vi "Facade.vi"(0 "Data In":T4, 2 "Display State In":T2, 3 "Container State":T3) -> (6 "Data Out":T4, 7 "Display State Out":T2, 8 "Action":T1)   [LabVIEW 2015, in "FM Sweep.xctl"]
uses:
  FM Sweep.xctl
  <vilib>/_xctls/Action.ctl
  <vilib>/_xctls/XControlSupport.lvlib
  Classes/Waveforms/FM Sweep/FM Sweep.lvclass
  <vilib>/_xctls/Container State.ctl
  Data.vi
  State.vi
panel:
  in  "mode":enum16{"Linear", "Log"}(ring)
  in  "ramp constant":bool caption="Hold freq const during ramp"
  in  "Fmax (Hz)":dbl
  in  "Fmin (Hz)":dbl
  in  "Rate":dbl caption="Rate (oct/s)"
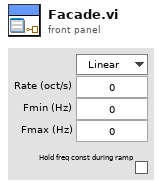
[diagram p1: front panel]
types:
  T1 = typedef "XControlSupport.lvlib/Action.ctl" = cluster{"Data Changed?":bool, "State Changed?":bool, "Action Name":string}
  T2 = typedef "FM Sweep.xctl/State.vi" = cluster{"Numeric":dbl}
  T3 = typedef "XControlSupport.lvlib/Container State.ctl" = cluster{"Indicator?":bool, "Run Mode?":bool, " Refnum":refnum<vi>}
  T4 = typedef "FM Sweep.xctl/Data.vi" = refnum<class "FM Sweep.lvclass">
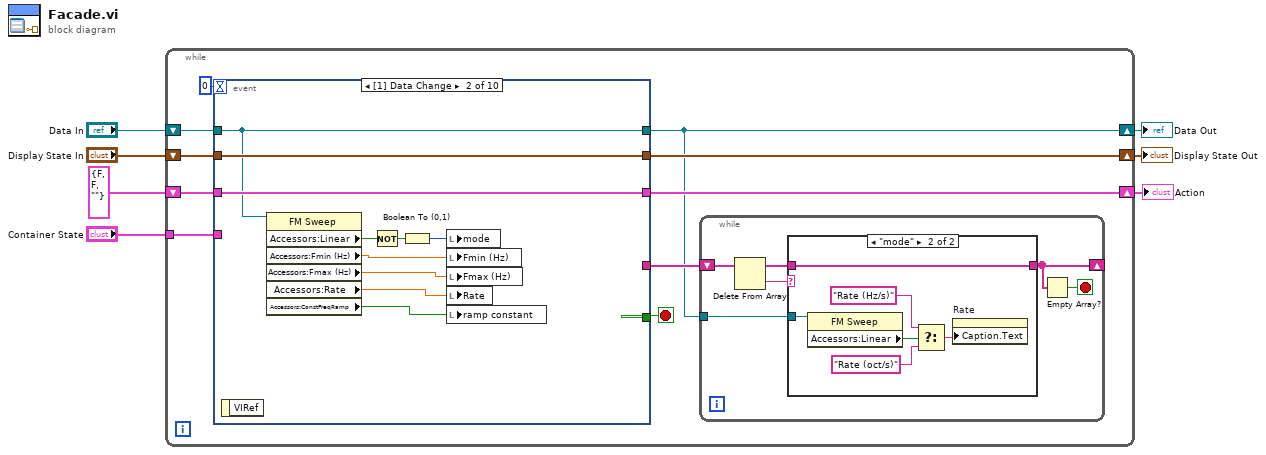
[diagram p0: block diagram]
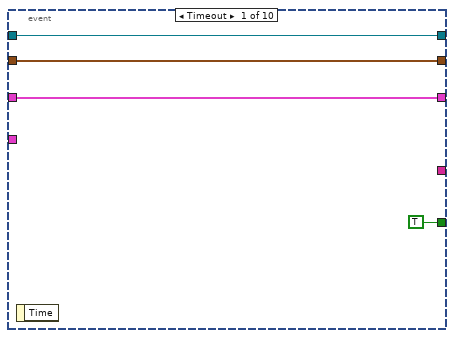
[diagram p3: hidden frame]
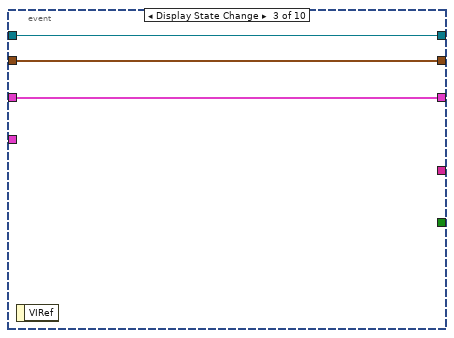
[diagram p4: hidden frame]
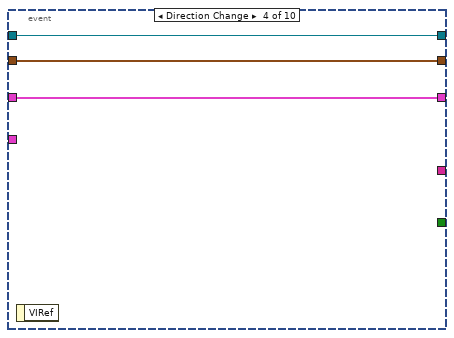
[diagram p5: hidden frame]
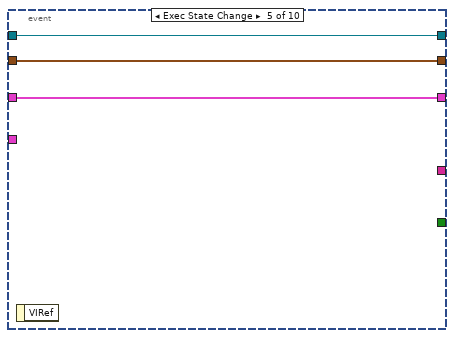
[diagram p6: hidden frame]
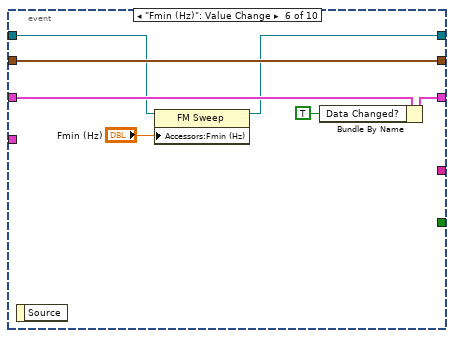
[diagram p7: hidden frame]
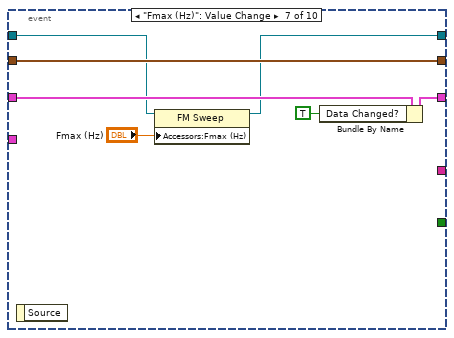
[diagram p8: hidden frame]
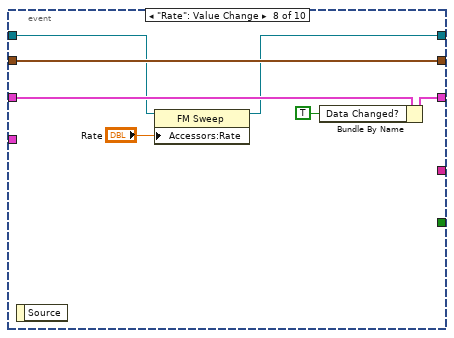
[diagram p9: hidden frame]
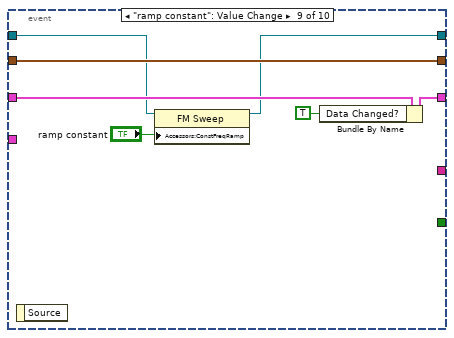
[diagram p10: hidden frame]
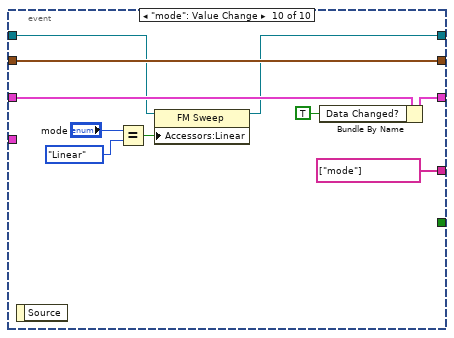
[diagram p11: hidden frame]
diagram:
  n1 = while {
    shift-right: [w16] -> w4
    shift-left: "Display State In" -> [w17]
    tunnel: "Container State" -> [w13]
    shift-right: [w8] -> w7
    shift-left: "Data In" -> [w12]
    shift-right: [w10] -> w2
    shift-left: T1 {"Data Changed?"=FALSE, "State Changed?"=FALSE, "Action Name"=""} ("Action") -> [w11]
    stop <- w15 stop-if-true
    n2 = event shown="[1] Data Change" {
      selector: _ -> [_ _ _ _ _ _ _ _ _ _]
      dyn-events: _ -> [_ _ _ _ _ _ _ _ _ _]
      timeout: 0 -> [_ _ _ _ _ _ _ _ _ _]
      tunnel: w17 -> [w32 w44 w47 w50 w53 w60 w67 w74 w81 w91]
      tunnel: [w32 w44 w47 w50 w53 w60 w67 w74 w81 w91] -> w16
      tunnel: [TRUE _ _ _ _ _ _ _ _ _] -> w15
      tunnel: w13 -> [_ _ _ _ _ _ _ _ _ _]
      tunnel: w12 -> [w31 w42 w46 w49 w52 w58 w65 w72 w79 w89]
      tunnel: [w31 w42 w46 w49 w52 w57 w64 w71 w78 w88] -> w8
      tunnel: [w33 w43 w45 w48 w51 w56 w63 w70 w77 w87] -> w10
      tunnel: w11 -> [w33 w43 w45 w48 w51 w59 w66 w73 w80 w90]
      tunnel: [_ _ _ _ _ _ _ _ _ string[] ["mode"]] -> w9
      event Timeout {
        n3 = event-data() -> ()  [unwired: 1 in, 1 out]
      }
      event Data Change {
        n4 = event-data() -> ()  [unwired: 1 in, 1 out]
        n5 = property class="FM Sweep"(reference=w42) -> ("Accessors:Linear"=w41:bool, "Accessors:Fmin (Hz)"=w38:dbl, "Accessors:Fmax (Hz)"=w37:dbl, "Accessors:Rate"=w36:dbl, "Accessors:ConstFreqRamp"=w35:bool)  [unwired: 1 in, 2 out]
        n6 = Not(x=w41) -> (.not. x?=w40:bool)
        n7 = Boolean To (0,1)(Boolean=w40) -> (0, 1=w39:i16)
        n8 = local write "mode"(w39) -> ()
        n9 = local write "Fmin (Hz)"(w38) -> ()
        n10 = local write "Fmax (Hz)"(w37) -> ()
        n11 = local write "Rate"(w36) -> ()
        n12 = local write "ramp constant"(w35) -> ()
      }
      event Display State Change {
        n13 = event-data() -> ()  [unwired: 1 in, 1 out]
      }
      event Direction Change {
        n14 = event-data() -> ()  [unwired: 1 in, 1 out]
      }
      event Exec State Change {
        n15 = event-data() -> ()  [unwired: 1 in, 1 out]
      }
      event "Fmin (Hz)": Value Change {
        n16 = event-data() -> ()  [unwired: 1 in, 1 out]
        n17 = property class="FM Sweep"(reference=w58, "Accessors:Fmin (Hz)"="Fmin (Hz)") -> (reference out=w57:T4)  [unwired: 1 in, 1 out]
        n18 = Bundle By Name(cluster=w59, "Data Changed?"=TRUE) -> (w56:T1)
      }
      event "Fmax (Hz)": Value Change {
        n19 = event-data() -> ()  [unwired: 1 in, 1 out]
        n20 = property class="FM Sweep"(reference=w65, "Accessors:Fmax (Hz)"="Fmax (Hz)") -> (reference out=w64:T4)  [unwired: 1 in, 1 out]
        n21 = Bundle By Name(cluster=w66, "Data Changed?"=TRUE) -> (w63:T1)
      }
      event "Rate": Value Change {
        n22 = event-data() -> ()  [unwired: 1 in, 1 out]
        n23 = property class="FM Sweep"(reference=w72, "Accessors:Rate"="Rate") -> (reference out=w71:T4)  [unwired: 1 in, 1 out]
        n24 = Bundle By Name(cluster=w73, "Data Changed?"=TRUE) -> (w70:T1)
      }
      event "ramp constant": Value Change {
        n25 = event-data() -> ()  [unwired: 1 in, 1 out]
        n26 = property class="FM Sweep"(reference=w79, "Accessors:ConstFreqRamp"="ramp constant") -> (reference out=w78:T4)  [unwired: 1 in, 1 out]
        n27 = Bundle By Name(cluster=w80, "Data Changed?"=TRUE) -> (w77:T1)
      }
      event "mode": Value Change {
        n28 = event-data() -> ()  [unwired: 1 in, 1 out]
        n29 = Equal?(x="mode", y=enum16{"Linear", "Log"}."Linear") -> (x = y?=w83:bool)
        n30 = property class="FM Sweep"(reference=w89, "Accessors:Linear"=w83) -> (reference out=w88:T4)  [unwired: 1 in, 1 out]
        n31 = Bundle By Name(cluster=w90, "Data Changed?"=TRUE) -> (w87:T1)
      }
    }
    n32 = while {
      shift-right: [w20] -> _
      shift-left: w9 -> [w23]
      tunnel: w8 -> [w18]
      stop <- w19 stop-if-true
      n33 = Delete From Array(array=w23) -> (deleted portion=w21:string, array with subset deleted=w22:string[])  [unwired: 2 in]
      n34 = case shown="\"mode\"" w21 {
        tunnel: w22 -> [w24 w30]
        tunnel: [w24 w30] -> w20
        tunnel: w18 -> [_ w29]
        frame "", Default {
        }
        frame "mode" {
          n35 = property class="FM Sweep"(reference=w29) -> ("Accessors:Linear"=w28:bool)  [unwired: 1 in, 2 out]
          n36 = Select(t="Rate (Hz/s)", s=w28, f="Rate (oct/s)") -> (s? t:f=w27:string)
          n37 = property on="Rate" class="DigNum (strict)"("Caption.Text"=w27) -> ()  [unwired: 2 in, 2 out]
        }
      }
      n38 = Empty Array?(array=w20) -> (empty?=w19:bool)
    }
  }
  "Display State Out" <- w4
  "Data Out" <- w7
  "Action" <- w2
